vi "Module Initial State.vi"(8 "error in (no error)":errorcluster, 11 "launcher in":refnum<class "launcher.lvclass">) -> (0 "error out":errorcluster, 3 "launcher out":refnum<class "launcher.lvclass">)   [LabVIEW 2021, in "launcher.lvclass"]
uses:
  launcher.lvclass
  C:/Program Files (x86)/National Instruments/LabVIEW 2021/user.lib/S2 Labs/Module Framework/Modules/Base/Module.lvclass
  <userlib>/S2 Labs/Module Framework/Modules/Base/Module.lvclass/Module.ctl
  <userlib>/S2 Labs/Module Framework/Modules/Base/Write Logging Queue.vi
  <userlib>/S2 Labs/Module Framework/Modules/Base/Module.lvclass
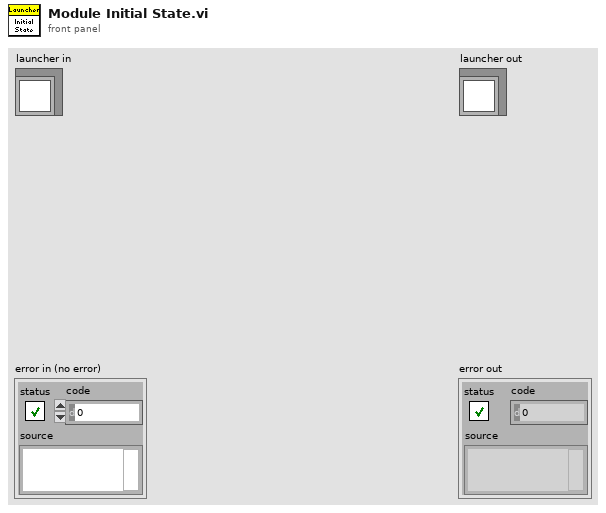
[diagram p1: front panel]
types:
  T1 = cluster{"Module":string, "Data Map":map{string, cluster{"value":dbl, "ts":timestamp, "variant":variant, "variant value?":bool}}}
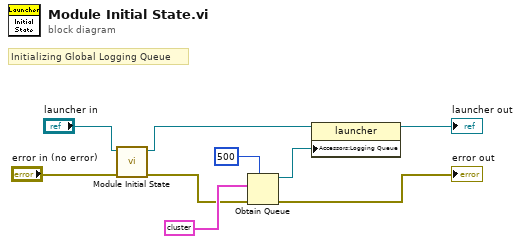
[diagram p0: block diagram]
diagram:
  # "Initializing Global Logging Queue"
  n1 = call-parent "Module Initial State.vi"("error in (no error)"="error in (no error)", "Module in"="launcher in") -> ("error out"=w5:errorcluster, "Module out"=w3:refnum<class "launcher.lvclass">)  [unwired: 8 in]
  n2 = Obtain Queue(max queue size (-1, unlimited)=500, element data type=T1 {"Module"="", "Data Map"={}} ("Data"), error in (no error)=w5) -> (queue out=w1:refnum<queue>, error out=→"error out":errorcluster)  [unwired: 2 in, 1 out]
  n3 = property class="launcher"(reference=w3, "Accessors:Logging Queue"=w1) -> (reference out=→"launcher out":refnum<class "launcher.lvclass">)  [unwired: 1 in, 1 out]
